vi "多个参数加标回收启动器.vi"(10 "流程":T1, 11 "启用参数选择":T2) -> ()   [LabVIEW 2016, in "质控单元V1.lvlib"]
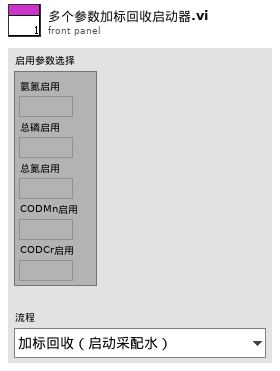
[diagram p1: front panel]
types:
  T1 = typedef "质控单元V1.lvlib/测试流程.ctl" = enum16{"加标回收（启动采配水）", "加标回收（不启动采配水）", "水样测试（启动采配水）", "水样测试（不启动采配水）", "平行样测试（启动采配水）", "平行样测试（不启动采配水）", "集成干预测试"}
  T2 = cluster{"氨氮启用":bool, "总磷启用":bool, "总氮启用":bool, "CODMn启用":bool, "CODCr启用":bool}
  T3 = typedef "质控单元V1.lvlib/测试子流程.ctl" = enum16{"水样测试（不启动采配水）", "水样测试（不含采样杯）", "加标回收（润洗采样合并）", "加标回收（不启动采配水）", "平行样测试（不启动采配水）", "平行样测试（不含采样杯）", "集成干预测试（不含采样杯）"}
  T4 = cluster{"氨氮":bool, "总磷":bool, "总氮":bool, "CODMn":bool, "CODCr":bool}
  T5 = typedef "质控单元V1.lvlib/质控slave id.ctl" = enum16{"null", "氨氮", "总磷", "CODMn", "CODCr", "总氮"}
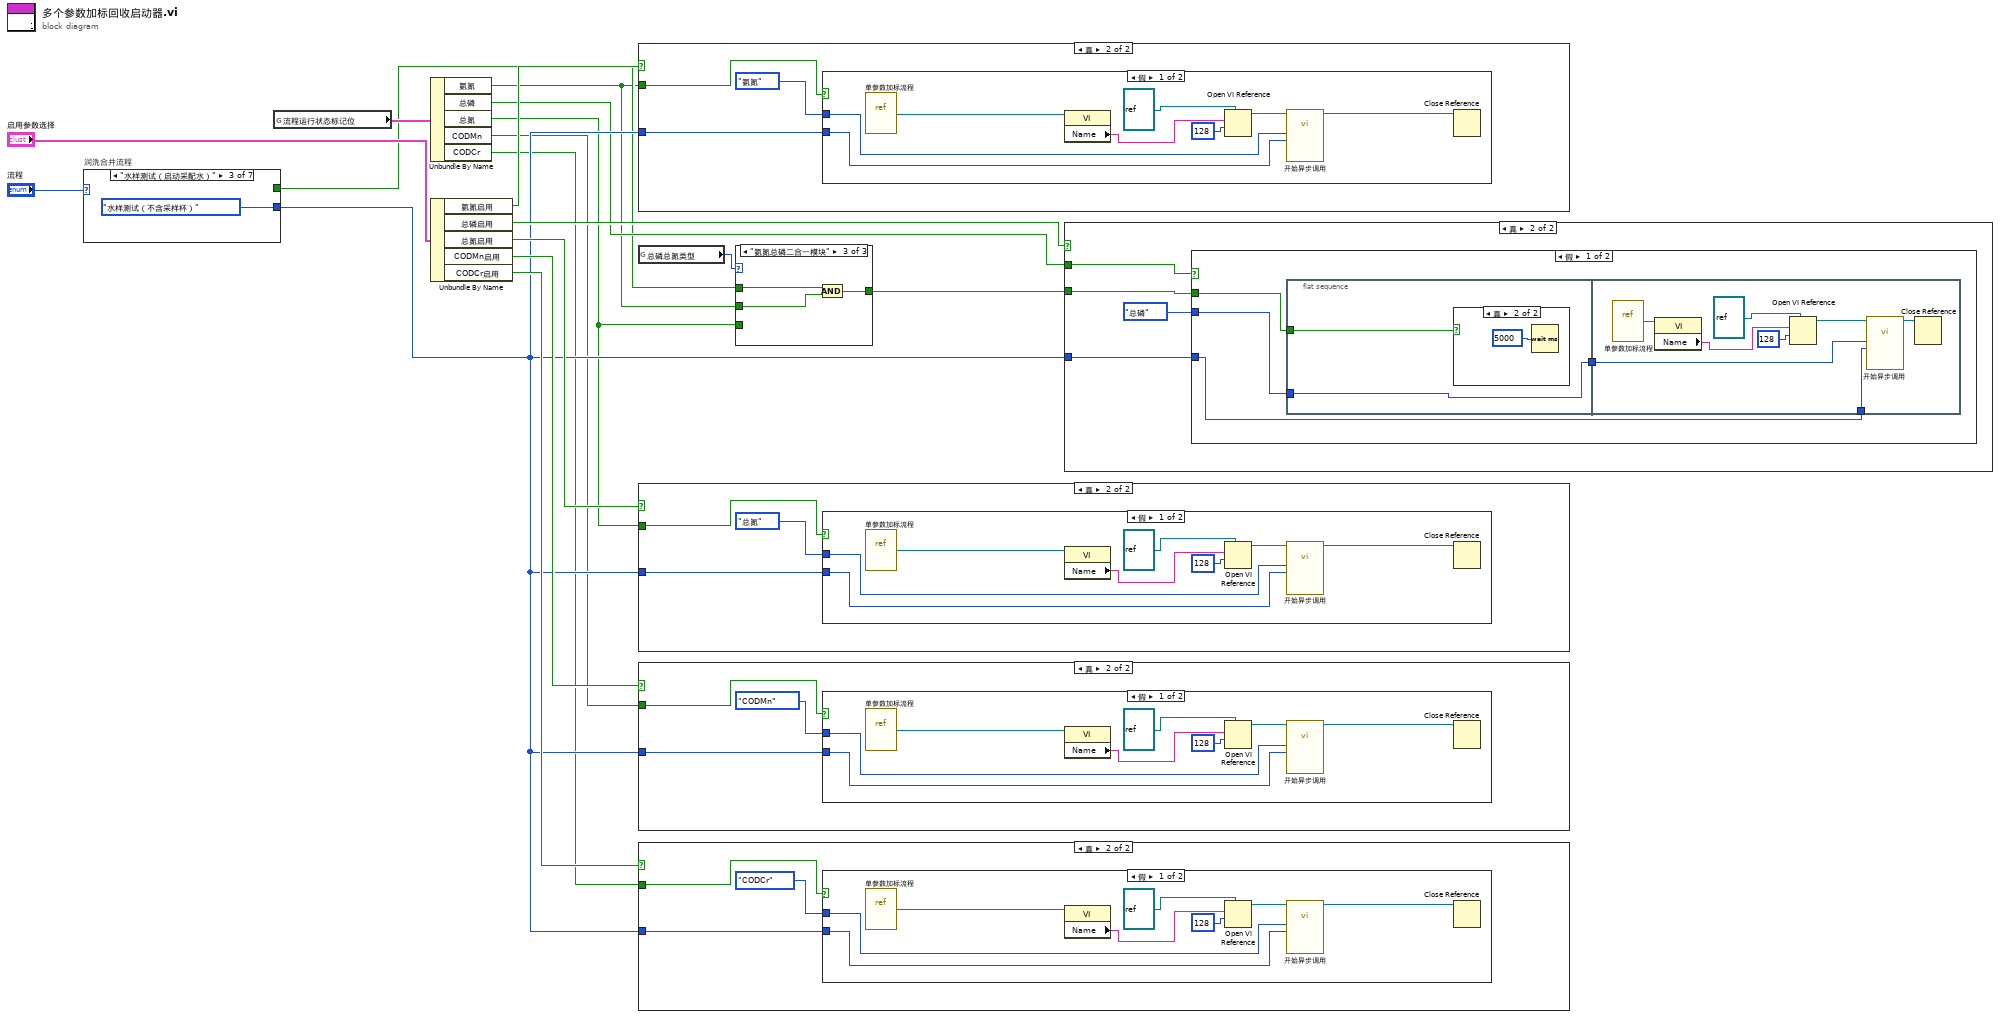
[diagram p0: block diagram]
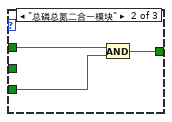
[diagram p3: hidden frame]
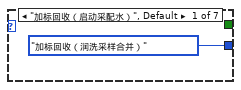
[diagram p4: hidden frame]
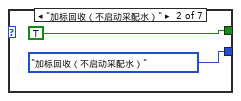
[diagram p5: hidden frame]
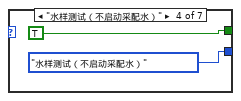
[diagram p6: hidden frame]
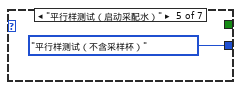
[diagram p7: hidden frame]
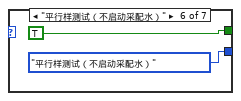
[diagram p8: hidden frame]
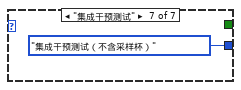
[diagram p9: hidden frame]
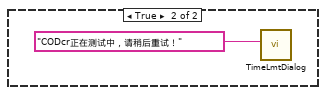
[diagram p11: hidden frame]
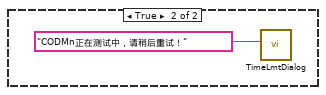
[diagram p13: hidden frame]
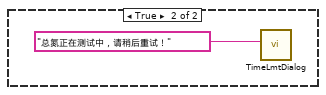
[diagram p15: hidden frame]
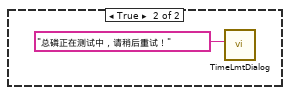
[diagram p18: hidden frame]
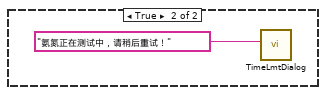
[diagram p20: hidden frame]
diagram:
  n1 = case "润洗合并流程" shown="\"水样测试（启动采配水）\"" "流程" {
    tunnel: [测试子流程."加标回收（润洗采样合并）" ("流程类型") 测试子流程."加标回收（不启动采配水）" ("流程类型") 测试子流程."水样测试（不含采样杯）" ("流程类型") 测试子流程."水样测试（不启动采配水）" ("流程类型") 测试子流程."平行样测试（不含采样杯）" ("流程类型") 测试子流程."平行样测试（不启动采配水）" ("流程类型") 测试子流程."集成干预测试（不含采样杯）" ("流程类型")] -> w10
    tunnel: [_ TRUE _ TRUE _ TRUE _] -> w4
    frame "加标回收（启动采配水）", Default {
    }
    frame "加标回收（不启动采配水）" {
    }
    frame "水样测试（启动采配水）" {
    }
    frame "水样测试（不启动采配水）" {
    }
    frame "平行样测试（启动采配水）" {
    }
    frame "平行样测试（不启动采配水）" {
    }
    frame "集成干预测试" {
    }
  }
  n2 = global read "ZK非断电保存全局变量.vi" "流程运行状态标记位"() -> (w9:T4)
  n3 = Unbundle By Name(w9) -> ("氨氮"=w2:bool, "总磷"=w8:bool, "总氮"=w3:bool, "CODMn"=w7:bool, "CODCr"=w6:bool)
  n4 = Unbundle By Name("启用参数选择") -> ("氨氮启用"=w16:bool, "总磷启用"=w15:bool, "总氮启用"=w14:bool, "CODMn启用"=w13:bool, "CODCr启用"=w12:bool)
  n5 = case shown="真" w16 {
    tunnel: w10 -> [_ w30]
    tunnel: w2 -> [_ w29]
    frame False {
    }
    frame True {
      n6 = case shown="假" w29 {
        tunnel: w30 -> [w32 _]
        tunnel: 质控slave_id."氨氮" ("Slave ID") -> [w33 _]
        frame False {
          n7 = vi-ref "单参数加标流程.vi"() -> (w34:refnum<vi>)
          n8 = property class="VI"(reference=w34) -> ("Name"=w35:string)  [unwired: 1 in, 2 out]
          n9 = Open VI Reference(type specifier VI Refnum (for type only)=refnum<vi> refnum, vi path=w35, options=128 ("选项")) -> (vi reference=w37:refnum<vi>)  [unwired: 3 in, 1 out]
          n10 = call-by-ref "开始异步调用"(reference=w37, "流程类型"=w32, "Slave ID"=w33) -> (reference out=w38:refnum<vi>)  [unwired: 11 in, 1 out]
          n11 = Close Reference(reference=w38) -> ()  [unwired: 1 in, 1 out]
        }
        frame True {
          n12 = call "TimeLmtDialog.vi"("Infoin"="氨氮正在测试中，请稍后重试！" ("消息")) -> ()  [unwired: 11 in]
        }
      }
    }
  }
  n13 = global read "系统交互.vi" "总磷总氮类型"() -> (w5:enum16{"单模块", "总磷总氮二合一模块", "氨氮总磷二合一模块"})
  n14 = case shown="真" w14 {
    tunnel: w10 -> [_ w41]
    tunnel: w3 -> [_ w40]
    frame False {
    }
    frame True {
      n15 = case shown="假" w40 {
        tunnel: w41 -> [w44 _]
        tunnel: 质控slave_id."总氮" ("Slave ID") -> [w45 _]
        frame False {
          n16 = vi-ref "单参数加标流程.vi"() -> (w46:refnum<vi>)
          n17 = property class="VI"(reference=w46) -> ("Name"=w47:string)  [unwired: 1 in, 2 out]
          n18 = Open VI Reference(type specifier VI Refnum (for type only)=refnum<vi> refnum, vi path=w47, options=128 ("选项")) -> (vi reference=w49:refnum<vi>)  [unwired: 3 in, 1 out]
          n19 = call-by-ref "开始异步调用"(reference=w49, "流程类型"=w44, "Slave ID"=w45) -> (reference out=w50:refnum<vi>)  [unwired: 11 in, 1 out]
          n20 = Close Reference(reference=w50) -> ()  [unwired: 1 in, 1 out]
        }
        frame True {
          n21 = call "TimeLmtDialog.vi"("Infoin"="总氮正在测试中，请稍后重试！" ("消息")) -> ()  [unwired: 11 in]
        }
      }
    }
  }
  n22 = case shown="真" w13 {
    tunnel: w10 -> [_ w52]
    tunnel: w7 -> [_ w53]
    frame False {
    }
    frame True {
      n23 = case shown="假" w53 {
        tunnel: w52 -> [w57 _]
        tunnel: 质控slave_id."CODMn" ("Slave ID") -> [w56 _]
        frame False {
          n24 = vi-ref "单参数加标流程.vi"() -> (w58:refnum<vi>)
          n25 = property class="VI"(reference=w58) -> ("Name"=w59:string)  [unwired: 1 in, 2 out]
          n26 = Open VI Reference(type specifier VI Refnum (for type only)=refnum<vi> refnum, vi path=w59, options=128 ("选项")) -> (vi reference=w61:refnum<vi>)  [unwired: 3 in, 1 out]
          n27 = call-by-ref "开始异步调用"(reference=w61, "流程类型"=w57, "Slave ID"=w56) -> (reference out=w62:refnum<vi>)  [unwired: 11 in, 1 out]
          n28 = Close Reference(reference=w62) -> ()  [unwired: 1 in, 1 out]
        }
        frame True {
          n29 = call "TimeLmtDialog.vi"("Infoin"="CODMn正在测试中，请稍后重试！" ("消息")) -> ()  [unwired: 11 in]
        }
      }
    }
  }
  n30 = case shown="真" w12 {
    tunnel: w10 -> [_ w64]
    tunnel: w6 -> [_ w65]
    frame False {
    }
    frame True {
      n31 = case shown="假" w65 {
        tunnel: w64 -> [w68 _]
        tunnel: 质控slave_id."CODCr" ("Slave ID") -> [w69 _]
        frame False {
          n32 = vi-ref "单参数加标流程.vi"() -> (w70:refnum<vi>)
          n33 = property class="VI"(reference=w70) -> ("Name"=w71:string)  [unwired: 1 in, 2 out]
          n34 = Open VI Reference(type specifier VI Refnum (for type only)=refnum<vi> refnum, vi path=w71, options=128 ("选项")) -> (vi reference=w73:refnum<vi>)  [unwired: 3 in, 1 out]
          n35 = call-by-ref "开始异步调用"(reference=w73, "流程类型"=w68, "Slave ID"=w69) -> (reference out=w74:refnum<vi>)  [unwired: 11 in, 1 out]
          n36 = Close Reference(reference=w74) -> ()  [unwired: 1 in, 1 out]
        }
        frame True {
          n37 = call "TimeLmtDialog.vi"("Infoin"="CODcr正在测试中，请稍后重试！" ("消息")) -> ()  [unwired: 11 in]
        }
      }
    }
  }
  n38 = case shown="\"氨氮总磷二合一模块\"" w5 {
    tunnel: w4 -> [_ w77 w81]
    tunnel: w3 -> [_ w78 _]
    tunnel: [_ w76 w80] -> w1
    tunnel: w2 -> [_ _ w79]
    frame "单模块", Default {
    }
    frame "总磷总氮二合一模块" {
      n39 = And(x=w77, y=w78) -> (x .and. y?=w76:bool)
    }
    frame "氨氮总磷二合一模块" {
      n40 = And(x=w81, y=w79) -> (x .and. y?=w80:bool)
    }
  }
  n41 = case shown="真" w15 {
    tunnel: w10 -> [_ w84]
    tunnel: w8 -> [_ w83]
    tunnel: w1 -> [_ w82]
    frame False {
    }
    frame True {
      n42 = case shown="假" w83 {
        tunnel: w84 -> [w89 _]
        tunnel: 质控slave_id."总磷" ("Slave ID") -> [w88 _]
        tunnel: w82 -> [w86 _]
        frame False {
          n43 = flat-sequence {
            tunnel: w88 -> [w91]
            tunnel: [w91] -> w87
            tunnel: w86 -> [w90]
            tunnel: w89 -> [w100]
            tunnel: w87 -> [w99]
            frame #0 {
              n44 = case shown="真" w90 {
                frame False {
                }
                frame True {
                  n45 = Wait (ms)(milliseconds to wait=u32 5000 ("等待时间（毫秒）")) -> ()  [unwired: 1 out]
                }
              }
            }
            frame #1 {
              n46 = vi-ref "单参数加标流程.vi"() -> (w95:refnum<vi>)
              n47 = property class="VI"(reference=w95) -> ("Name"=w96:string)  [unwired: 1 in, 2 out]
              n48 = Open VI Reference(type specifier VI Refnum (for type only)=refnum<vi> refnum, vi path=w96, options=128 ("选项")) -> (vi reference=w94:refnum<vi>)  [unwired: 3 in, 1 out]
              n49 = call-by-ref "开始异步调用"(reference=w94, "流程类型"=w100, "Slave ID"=w99) -> (reference out=w98:refnum<vi>)  [unwired: 11 in, 1 out]
              n50 = Close Reference(reference=w98) -> ()  [unwired: 1 in, 1 out]
            }
          }
        }
        frame True {
          n51 = call "TimeLmtDialog.vi"("Infoin"="总磷正在测试中，请稍后重试！" ("消息")) -> ()  [unwired: 11 in]
        }
      }
    }
  }
